vi "Solution_Lab2.vi"() -> ()   [LabVIEW 2011]
uses:
  <vilib>/measure/NI_MABase.lvlib
  <vilib>/Analysis/NI_AALBase.lvlib
panel:
  in  "phase":dbl(knob) scale=0.0..90.0
  out "DSB-SC Ratio":dbl
  out "Conv DSB Ratio":dbl
  out "Conv DSB Demo AM Time 3":dynamicdata(graph)
  out "DSB-SC Demo AM Time 2":dynamicdata(graph)
  out "DSB-SC AM Time":waveform(dbl)(graph)
  in  "stop":bool
  in  "Modulation Index":dbl(slide)=1.0 scale=0.0..1.0
  in  "Modullation Freq":dbl(slide)=10.0 scale=0.0..1000.0
  in  "Carrier Freq":dbl(knob)=10.0 scale=0.0..500000.0
  out "Conv DSB AM Time":waveform(dbl)(graph)
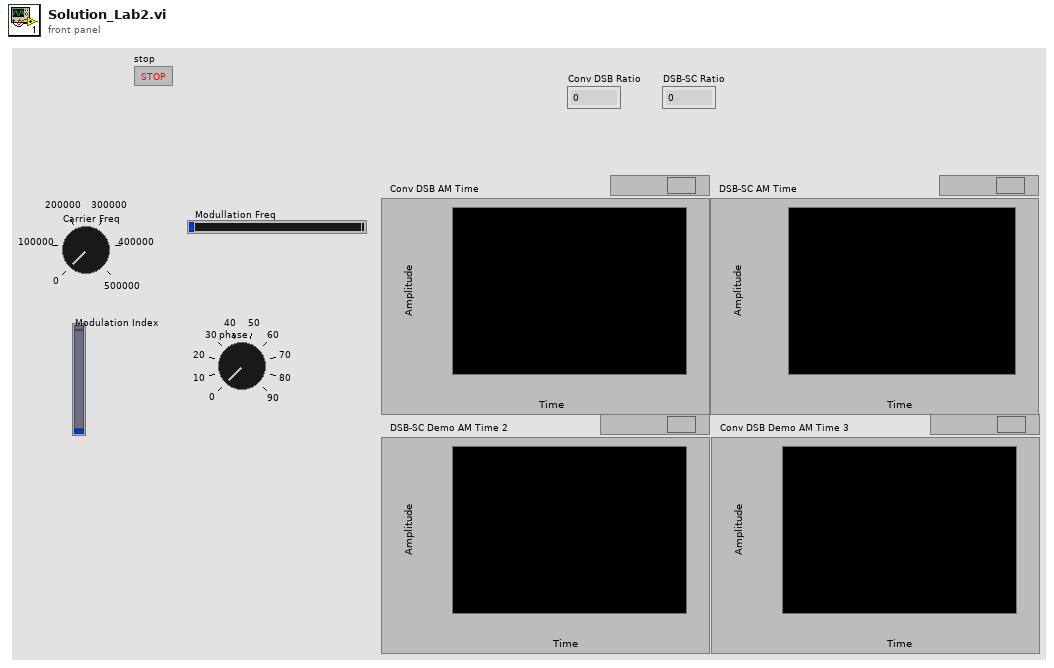
[diagram p1: front panel]
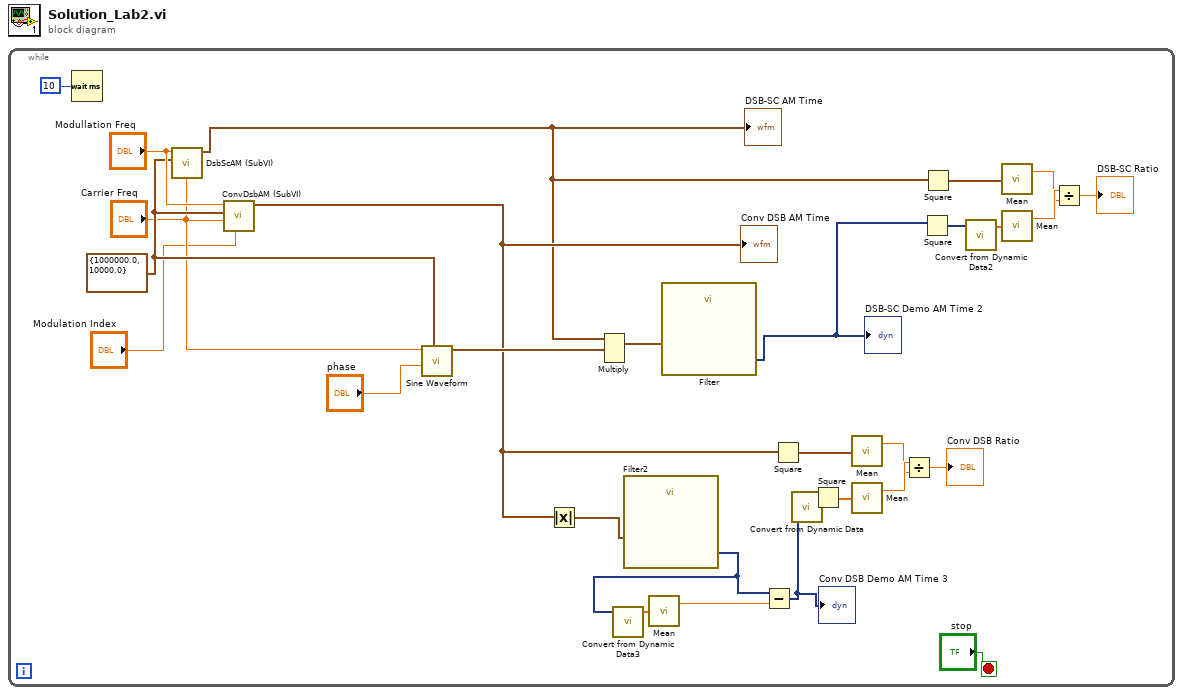
[diagram p0: block diagram]
diagram:
  n1 = while {
    stop <- "stop" stop-if-true
    w26 = cluster{"Fs":dbl, "#s":dbl} {"Fs"=1000000.0, "#s"=10000.0} ("sampling info")
    n2 = Wait (ms)(milliseconds to wait=u32 10) -> ()  [unwired: 1 out]
    n3 = call "DsbScAM (SubVI).vi"("Carrier Freq"="Carrier Freq", "sampling info"=w26, "Modulation Freq"="Modullation Freq") -> ("Waveform"=w6:waveform(dbl))  [unwired: 8 in]
    "DSB-SC AM Time" <- w6
    n4 = call "ConvDsbAM (SubVI).vi"("Modulation Index"="Modulation Index", "Carrier Freq"="Carrier Freq", "sampling info"=w26, "Modullation Freq"="Modullation Freq") -> ("Waveform"=w18:waveform(dbl))  [unwired: 7 in]
    "Conv DSB AM Time" <- w18
    n5 = call <vilib>:"Sine Waveform.vi"("sampling info"=w26, "phase"="phase", "frequency"="Carrier Freq") -> ("signal out"=w23:waveform(dbl))  [unwired: 7 in, 1 out]
    n6 = Absolute Value(x=w18) -> (abs(x)=w22:waveform(dbl))
    n7 = Multiply(1:w23, 2:w6) -> (0:w24:waveform(dbl))  [unwired: 1 in, 1 out]
    n8 = call "Filter2"("Signal"=w22) -> ("Filtered Signal"=w2:dynamicdata)  [unwired: 9 in, 1 out]
    n9 = call "Convert from Dynamic Data3"("Dynamic Data Type"=w2) -> ("Array"=w1:dbl[])  [unwired: 3 in]
    n10 = call <vilib>:"Mean.vi"("X"=w1) -> ("mean"=w21:dbl)  [unwired: 1 out]
    n11 = call "Filter"("Signal"=w24) -> ("Filtered Signal"=w9:dynamicdata)  [unwired: 9 in, 1 out]
    "DSB-SC Demo AM Time 2" <- w9
    n12 = Subtract(x=w2, y=w21) -> (x-y=w13:dynamicdata)
    "Conv DSB Demo AM Time 3" <- w13
    n13 = Square(x=w18) -> (x^2=w17:waveform(dbl))
    n14 = Square(x=w13) -> (x^2=w20:dynamicdata)
    n15 = call "Convert from Dynamic Data"("Dynamic Data Type"=w20) -> ("Array"=w19:dbl[])  [unwired: 3 in]
    n16 = call <vilib>:"Mean.vi"("X"=w17) -> ("mean"=w15:dbl)  [unwired: 1 out]
    n17 = call <vilib>:"Mean.vi"("X"=w19) -> ("mean"=w16:dbl)  [unwired: 1 out]
    n18 = Divide(x=w16, y=w15) -> (x/y=→"Conv DSB Ratio":dbl)
    n19 = Square(x=w9) -> (x^2=w8:dynamicdata)
    n20 = Square(x=w6) -> (x^2=w5:waveform(dbl))
    n21 = call "Convert from Dynamic Data2"("Dynamic Data Type"=w8) -> ("Array"=w7:dbl[])  [unwired: 3 in]
    n22 = call <vilib>:"Mean.vi"("X"=w5) -> ("mean"=w11:dbl)  [unwired: 1 out]
    n23 = call <vilib>:"Mean.vi"("X"=w7) -> ("mean"=w12:dbl)  [unwired: 1 out]
    n24 = Divide(x=w12, y=w11) -> (x/y=→"DSB-SC Ratio":dbl)
  }
